vi "User Event FGV.vi"(7 "Action":T1, 8 "error in (no error)":errorcluster) -> (0 "error out":errorcluster, 3 "Event Registration Refnum out":refnum<event-registration>)   [LabVIEW 2018, in "Queue Library.lvlib"]
uses:
  Queue Library.lvlib
  User Event Action Enum.ctl
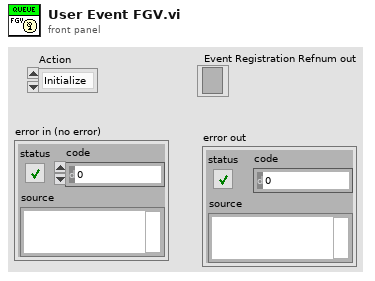
[diagram p1: front panel]
types:
  T1 = typedef "Queue Library.lvlib/User Event Action Enum.ctl" = enum16{"Initialize", "Generate", "Destroy"}
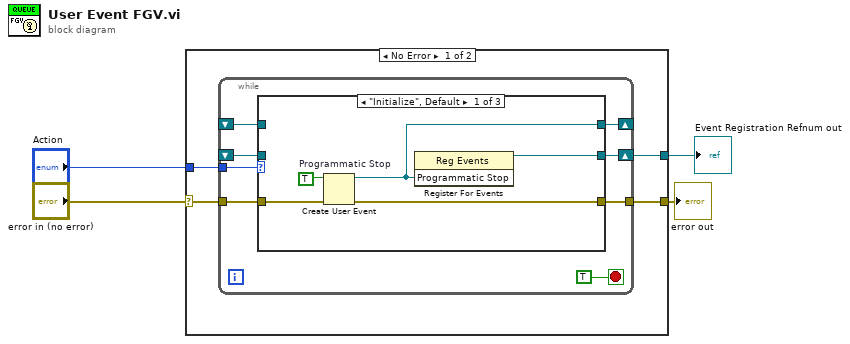
[diagram p0: block diagram]
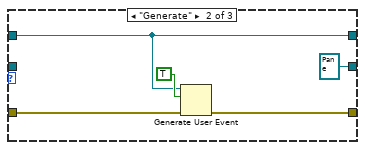
[diagram p2: hidden frame]
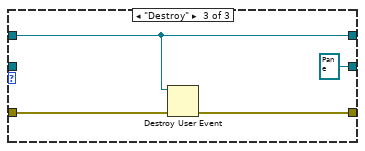
[diagram p3: hidden frame]
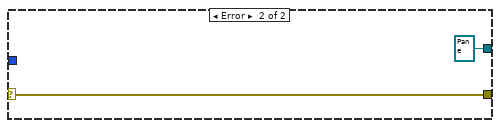
[diagram p4: hidden frame]
diagram:
  n1 = case shown="No Error" "error in (no error)" {
    selector: "error in (no error)" -> [w6 w32]
    tunnel: [w8 refnum<event-registration> refnum ("Event Registration Refnum")] -> w4
    tunnel: "Action" -> [w7 _]
    tunnel: [w5 w32] -> w1
    frame No Error {
      n2 = while {
        tunnel: w6 -> [w15]
        tunnel: w7 -> [w13]
        shift-right: [w16] -> w8
        shift-left: _ -> [w12]
        shift-right: [w11] -> _
        shift-left: _ -> [w10]
        tunnel: [w9] -> w5
        stop <- TRUE stop-if-true
        n3 = case shown="\"Initialize\", Default" w13 {
          tunnel: [w21 refnum<event-registration> refnum ("Event Registration Refnum") refnum<event-registration> refnum ("Event Registration Refnum")] -> w16
          tunnel: w15 -> [w20 w25 w30]
          tunnel: w12 -> [_ _ _]
          tunnel: [w18 w23 w29] -> w11
          tunnel: w10 -> [_ w23 w29]
          tunnel: [w17 w24 w28] -> w9
          frame "Initialize", Default {
            w19 = TRUE  # Programmatic Stop
            n4 = Create User Event(user event datatype=w19, error in=w20) -> (user event=w18:refnum<user-event>, error out=w17:errorcluster)
            n5 = register-events(w18) -> (reference out=w21:refnum<event-registration>)  [unwired: 2 in, 1 out]
          }
          frame "Generate" {
            n6 = Generate User Event(user event=w23, event data cluster=TRUE ("event data"), error in=w25) -> (error out=w24:errorcluster)  [unwired: 1 in, 1 out]
          }
          frame "Destroy" {
            n7 = Destroy User Event(user event=w29, error in=w30) -> (error out=w28:errorcluster)
          }
        }
      }
    }
    frame Error {
    }
  }
  "Event Registration Refnum out" <- w4
  "error out" <- w1
